vi "AutonDrive.vi"(5 "Stop Time":dbl, 7 "Drive Time":dbl, 9 "Right Input":dbl format="%#_13g", 10 "Left Input":dbl format="%#_13g") -> ()   [LabVIEW 2015]
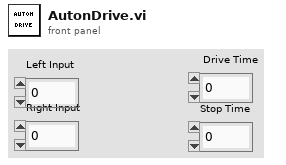
[diagram p1: front panel]
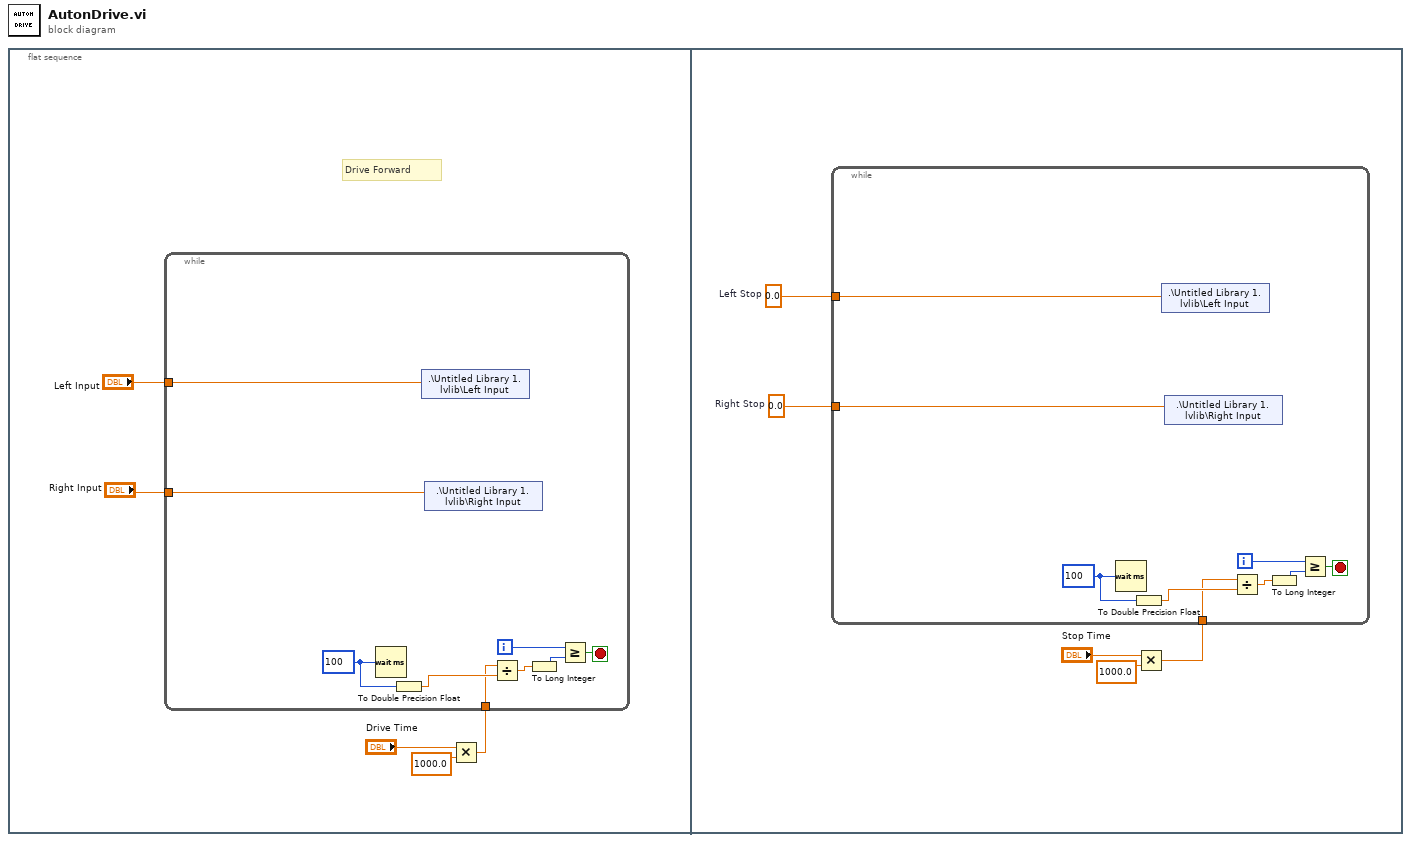
[diagram p0: block diagram]
diagram:
  n1 = flat-sequence {
    frame #0 {
      # "Drive Forward"
      n2 = Multiply(x="Drive Time", y=1000.0) -> (x*y=w5:dbl)
      n3 = while {
        tunnel: "Left Input" -> [w7]
        tunnel: "Right Input" -> [w6]
        tunnel: w5 -> [w8]
        i -> [w10]
        stop <- w9 stop-if-true
        w14 = u32 100 ("milliseconds to wait")
        n4 = Wait (ms)(milliseconds to wait=w14) -> ()  [unwired: 1 out]
        n5 = To Double Precision Float(number=w14) -> (double precision float=w13:dbl)
        n6 = shared-variable ".\\Untitled Library 1.lvlib\\Left Input"(w7) -> ()  [unwired: 1 in, 1 out]
        n7 = shared-variable ".\\Untitled Library 1.lvlib\\Right Input"(w6) -> ()  [unwired: 1 in, 1 out]
        n8 = Divide(x=w8, y=w13) -> (x/y=w12:dbl)
        n9 = To Long Integer(number=w12) -> (32bit integer=w11:i32)
        n10 = Greater Or Equal?(x=w10, y=w11) -> (x >= y?=w9:bool)
      }
    }
    frame #1 {
      w18 = 0.0  # Right Stop
      w19 = 0.0  # Left Stop
      n11 = Multiply(x="Stop Time", y=1000.0) -> (x*y=w15:dbl)
      n12 = while {
        tunnel: w19 -> [w20]
        tunnel: w18 -> [w21]
        tunnel: w15 -> [w22]
        i -> [w24]
        stop <- w23 stop-if-true
        w28 = u32 100 ("milliseconds to wait")
        n13 = Wait (ms)(milliseconds to wait=w28) -> ()  [unwired: 1 out]
        n14 = To Double Precision Float(number=w28) -> (double precision float=w27:dbl)
        n15 = shared-variable ".\\Untitled Library 1.lvlib\\Left Input"(w20) -> ()  [unwired: 1 in, 1 out]
        n16 = shared-variable ".\\Untitled Library 1.lvlib\\Right Input"(w21) -> ()  [unwired: 1 in, 1 out]
        n17 = Divide(x=w22, y=w27) -> (x/y=w26:dbl)
        n18 = To Long Integer(number=w26) -> (32bit integer=w25:i32)
        n19 = Greater Or Equal?(x=w24, y=w25) -> (x >= y?=w23:bool)
      }
    }
  }
